vi "ma_SML OBW (x dB method).vi"(8 "error in (no error)":errorcluster, 9 "x dB":dbl format="%.2f", 10 "spectral info in":T2 {"window" items=["Rectangle"=0, "Hanning"=1, "Hamming"=2, "Blackman-Harris"=3, "Exact Blackman"=4, "Blackman"=5, "Flat Top"=6, "4 Term B-Harris "=7, "7 Term B-Harris"=8, "Low Sidelobe"=9, "Blackman Nuttall"=11, "Triangle"=30, "Bartlett-Hanning"=31, "Bohman"=32, "Parzen"=33, "Welch"=34, "Kaiser"=60, "Dolph-Chebyshev"=61, "Gaussian"=62]}, 11 "power spectrum":T1={"f0"=0.0, "df"=1.0, "spectrum"=[]} {"spectrum" format="%.2f"; "df" format="%.2f"; "f0" format="%.2f"}) -> (0 "error out":errorcluster, 1 "fh [Hz]":dbl format="%.2f", 2 "fl [Hz]":dbl format="%.2f", 3 "occupied BW [Hz]":dbl format="%.2f")   [LabVIEW 2020, in "NI_MAPro.lvlib"]
uses:
  NI_MAPro.lvlib
  ma_sml_Spectral Info.ctl
  ma_sml_Spectrum Cluster (real).ctl
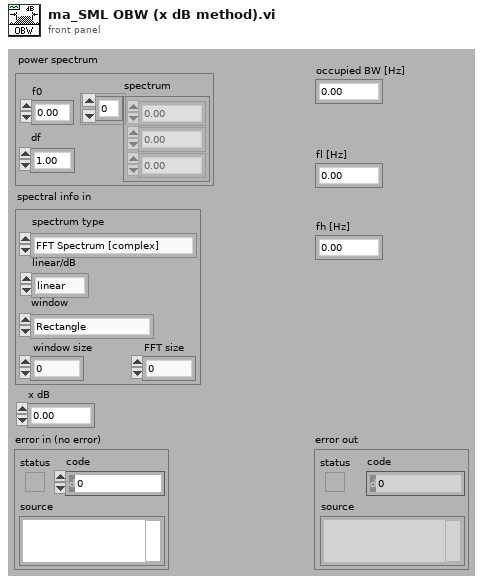
[diagram p1: front panel]
types:
  T1 = typedef "NI_MAPro.lvlib/ma_sml_Spectrum Cluster (real).ctl" = cluster{"f0":dbl, "df":dbl, "spectrum":dbl[]}
  T2 = typedef "NI_MAPro.lvlib/ma_sml_Spectral Info.ctl" = cluster{"spectrum type":enum16{"FFT Spectrum [complex]", "Amplitude [Magnitude]", "Power [Magnitude^2]", "Cross Spectrum [complex]", "Frequency Response [Complex]"}, "linear/dB":enum16{"linear", "dB"}, "window":u16, "window size":i32, "FFT size":i32}
  T3 = enum16{"FFT Spectrum [complex]", "Amplitude [Magnitude]", "Power [Magnitude^2]", "Cross Spectrum [complex]", "Frequency Response [Complex]"}
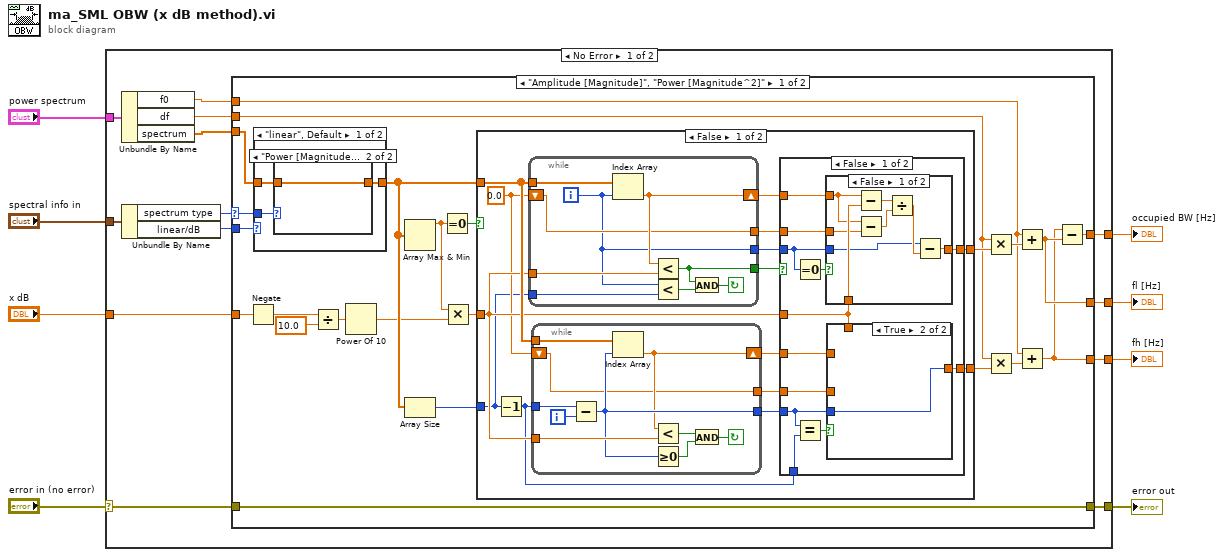
[diagram p0: block diagram]
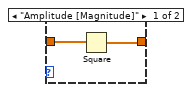
[diagram p2: hidden frame]
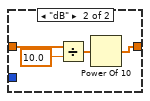
[diagram p3: hidden frame]
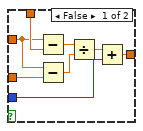
[diagram p4: hidden frame]
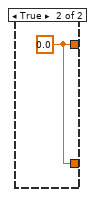
[diagram p6: hidden frame]
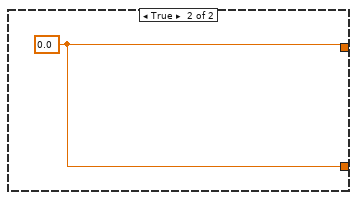
[diagram p7: hidden frame]
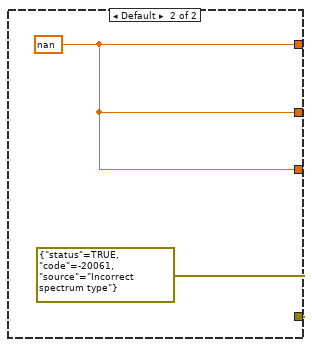
[diagram p8: hidden frame]
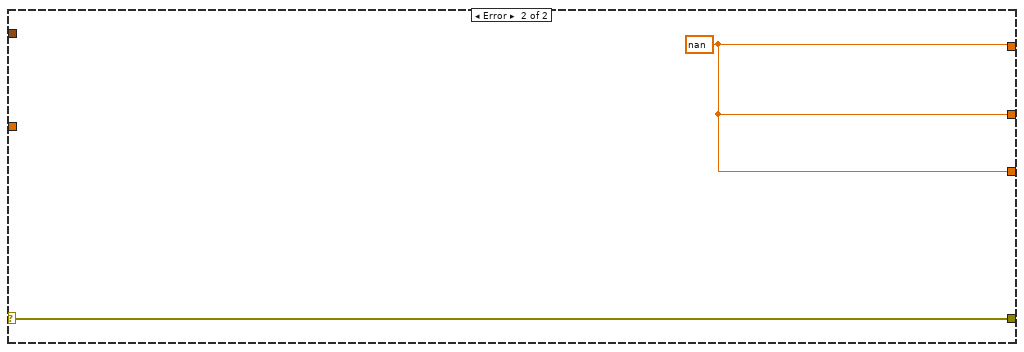
[diagram p9: hidden frame]
diagram:
  n1 = case shown="No Error" "error in (no error)" {
    selector: "error in (no error)" -> [w19 w123]
    tunnel: [w21 w123] -> w5
    tunnel: "x dB" -> [w20 _]
    tunnel: "power spectrum" -> [w18 _]
    tunnel: "spectral info in" -> [w15 _]
    tunnel: [w12 w122] -> w2
    tunnel: [w11 w122] -> w1
    tunnel: [w10 w122] -> w3
    frame No Error {
      n2 = Unbundle By Name(w18) -> ("f0"=w13:dbl, "df"=w14:dbl, "spectrum"=w17:dbl[])
      n3 = Unbundle By Name(w15) -> ("spectrum type"=w9:T3, "linear/dB"=w16:enum16{"linear", "dB"})
      n4 = case shown="\"Amplitude [Magnitude]\", \"Power [Magnitude^2]\"" w9 {
        selector: w9 -> [w36 _]
        tunnel: [w39 errorcluster {"status"=TRUE, "code"=-20061, "source"="Incorrect spectrum type"} ("error IO")] -> w21
        tunnel: w17 -> [w44 _]
        tunnel: w20 -> [w23 _]
        tunnel: w16 -> [w40 _]
        tunnel: w19 -> [w39 _]
        tunnel: w14 -> [w31 _]
        tunnel: w13 -> [w30 _]
        tunnel: [w29 w120] -> w12
        tunnel: [w28 w120] -> w11
        tunnel: [w27 w120] -> w10
        frame "Amplitude [Magnitude]", "Power [Magnitude^2]" {
          n5 = Negate(x=w23) -> (-x=w24:dbl)
          n6 = case shown="\"linear\", Default" w40 {
            tunnel: w36 -> [w47 _]
            tunnel: w44 -> [w46 w52]
            tunnel: [w45 w54] -> w38
            frame "linear", Default {
              n7 = case shown="\"Power [Magnitude^2]\", Default" w47 {
                tunnel: w46 -> [w49 w50]
                tunnel: [w48 w50] -> w45
                frame "Amplitude [Magnitude]" {
                  n8 = Square(x=w49) -> (x^2=w48:dbl[])
                }
                frame "Power [Magnitude^2]", Default {
                }
              }
            }
            frame "dB" {
              n9 = Divide(x=w52, y=10.0 ("Occupied BW [Hz]")) -> (x/y=w53:dbl[])
              n10 = Power Of 10(x=w53) -> (10^x=w54:dbl[])
            }
          }
          n11 = Divide(x=w24, y=10.0 ("Occupied BW [Hz]")) -> (x/y=w25:dbl)
          n12 = Power Of 10(x=w25) -> (10^x=w22:dbl)
          n13 = Array Max & Min(array=w38) -> (max value=w37:dbl)  [unwired: 3 out]
          n14 = Array Size(array=w38) -> (size(s)=w41:i32)
          n15 = Equal To 0?(x=w37) -> (x = 0?=w43:bool)
          n16 = Multiply(x=w37, y=w22) -> (x*y=w42:dbl)
          n17 = case shown="False" w43 {
            tunnel: [w67 w119] -> w33
            tunnel: [w66 w119] -> w32
            tunnel: w38 -> [w68 _]
            tunnel: w42 -> [w61 _]
            tunnel: w41 -> [w57 _]
            frame False {
              w60 = 0.0 ("Numeric")
              n18 = Decrement(x=w57) -> (x-1=w56:i32)
              n19 = while {
                tunnel: w61 -> [w107]
                tunnel: [w104] -> w59
                tunnel: w68 -> [w108]
                shift-right: [w106] -> w65
                shift-left: w60 -> [w105]
                tunnel: [w105] -> w64
                tunnel: w57 -> [w103]
                tunnel: [w100] -> w55
                i -> [w104]
                stop <- w102 continue-if-true
                n20 = Index Array(array=w108, index=w104) -> (element=w106:dbl)
                n21 = Less?(x=w106, y=w107) -> (x < y?=w100:bool)
                n22 = Less?(x=w104, y=w103) -> (x < y?=w101:bool)
                n23 = And(x=w100, y=w101) -> (x .and. y?=w102:bool)
              }
              n24 = while {
                tunnel: [w114] -> w58
                tunnel: w61 -> [w115]
                tunnel: w56 -> [w116]
                tunnel: w68 -> [w117]
                shift-right: [w113] -> w63
                shift-left: w60 -> [w110]
                tunnel: [w110] -> w62
                i -> [w118]
                stop <- w111 continue-if-true
                n25 = Subtract(x=w116, y=w118) -> (x-y=w114:i32)
                n26 = Index Array(array=w117, index=w114) -> (element=w113:dbl)
                n27 = Less?(x=w113, y=w115) -> (x < y?=w109:bool)
                n28 = Greater Or Equal To 0?(x=w114) -> (x >= 0?=w112:bool)
                n29 = And(x=w109, y=w112) -> (x .and. y?=w111:bool)
              }
              n30 = case shown="False" w55 {
                tunnel: [w80 w99] -> w67
                tunnel: [w79 w99] -> w66
                tunnel: w65 -> [w78 _]
                tunnel: w64 -> [w77 _]
                tunnel: w63 -> [w76 _]
                tunnel: w62 -> [w75 _]
                tunnel: w61 -> [w74 _]
                tunnel: w59 -> [w73 _]
                tunnel: w58 -> [w72 _]
                tunnel: w56 -> [w71 _]
                frame False {
                  n31 = Equal To 0?(x=w73) -> (x = 0?=w70:bool)
                  n32 = Equal?(x=w72, y=w71) -> (x = y?=w69:bool)
                  n33 = case shown="False" w70 {
                    tunnel: [w90 w98] -> w80
                    tunnel: w73 -> [w91 w98]
                    tunnel: w74 -> [w95 _]
                    tunnel: w78 -> [w94 _]
                    tunnel: w77 -> [w93 _]
                    frame False {
                      n34 = Subtract(x=w94, y=w95) -> (x-y=w97:dbl)
                      n35 = Subtract(x=w94, y=w93) -> (x-y=w92:dbl)
                      n36 = Divide(x=w97, y=w92) -> (x/y=w96:dbl)
                      n37 = Subtract(x=w91, y=w96) -> (x-y=w90:dbl)
                    }
                    frame True {
                    }
                  }
                  n38 = case shown="True" w69 {
                    tunnel: w74 -> [w88 _]
                    tunnel: [w82 w89] -> w79
                    tunnel: w72 -> [w81 w89]
                    tunnel: w76 -> [w84 _]
                    tunnel: w75 -> [w83 _]
                    frame False {
                      n39 = Subtract(x=w84, y=w88) -> (x-y=w87:dbl)
                      n40 = Subtract(x=w84, y=w83) -> (x-y=w85:dbl)
                      n41 = Divide(x=w87, y=w85) -> (x/y=w86:dbl)
                      n42 = Add(x=w86, y=w81) -> (x+y=w82:dbl)
                    }
                    frame True {
                    }
                  }
                }
                frame True {
                  w99 = 0.0
                }
              }
            }
            frame True {
              w119 = 0.0 ("Occupied BW [Hz]")
            }
          }
          n43 = Multiply(x=w31, y=w33) -> (x*y=w34:dbl)
          n44 = Multiply(x=w31, y=w32) -> (x*y=w35:dbl)
          n45 = Add(x=w30, y=w34) -> (x+y=w29:dbl)
          n46 = Add(x=w30, y=w35) -> (x+y=w28:dbl)
          n47 = Subtract(x=w28, y=w29) -> (x-y=w27:dbl)
        }
        frame Default {
          w120 = nan ("Occupied BW [Hz]")
        }
      }
    }
    frame Error {
      w122 = nan ("Occupied BW [Hz]")
    }
  }
  "error out" <- w5
  "occupied BW [Hz]" <- w3
  "fl [Hz]" <- w2
  "fh [Hz]" <- w1
